vi "CustomPID_v2.1.vi"(0 "Kp":dbl, 1 "Process Variable":dbl, 2 "Goal":dbl, 5 "Ki":dbl, 7 "Kd":dbl, 9 "N-Diff":i32=3, 11 "N-Int":i32=12, 12 "Reinit":bool, 13 "Max Ouput":dbl=1.0, 14 "Min Output":dbl=-1.0) -> (4 "Current Error":dbl, 8 "Command":dbl, 15 "PID Tracking":T1(graph))   [LabVIEW 2016]
uses:
  <vilib>/Analysis/NI_AALPro.lvlib
panel:
  out "x-y":u32
  out "Absolute Iterations":i32
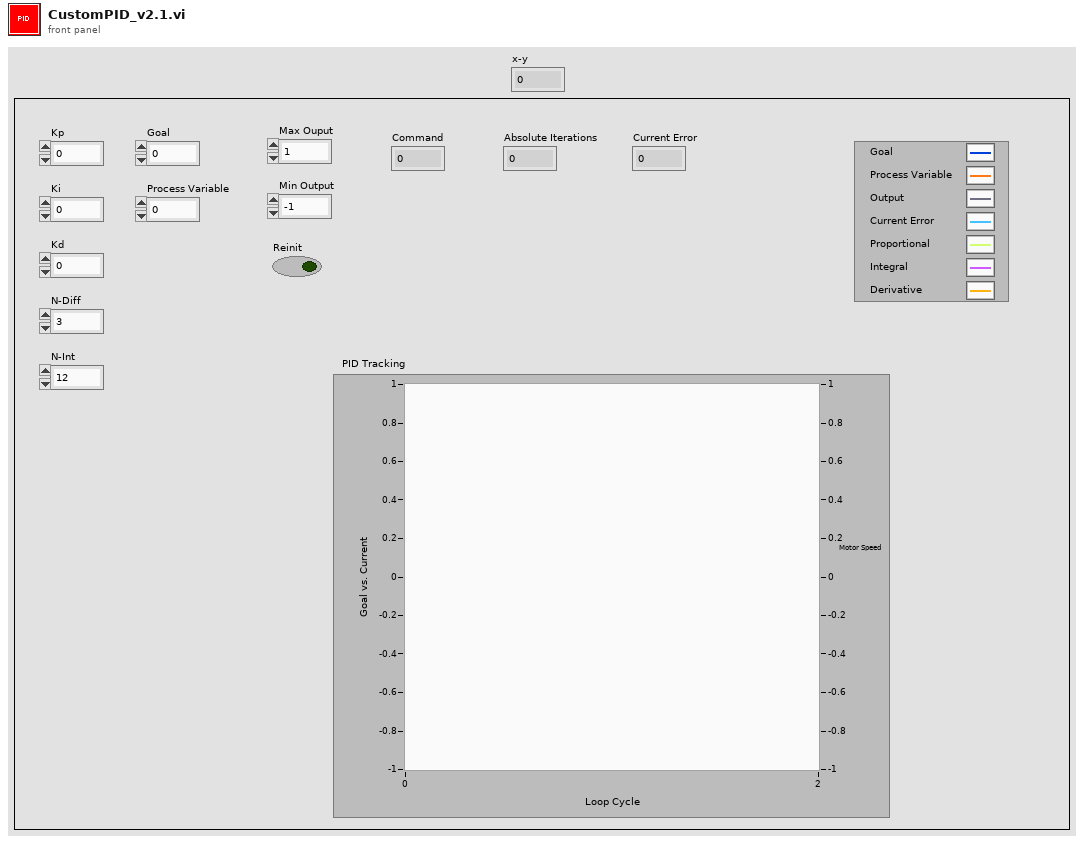
[diagram p1: front panel]
types:
  T1 = cluster{"Goal":dbl, "Process Variable":dbl, "Max Ouput":dbl, dbl, dbl, dbl, dbl}
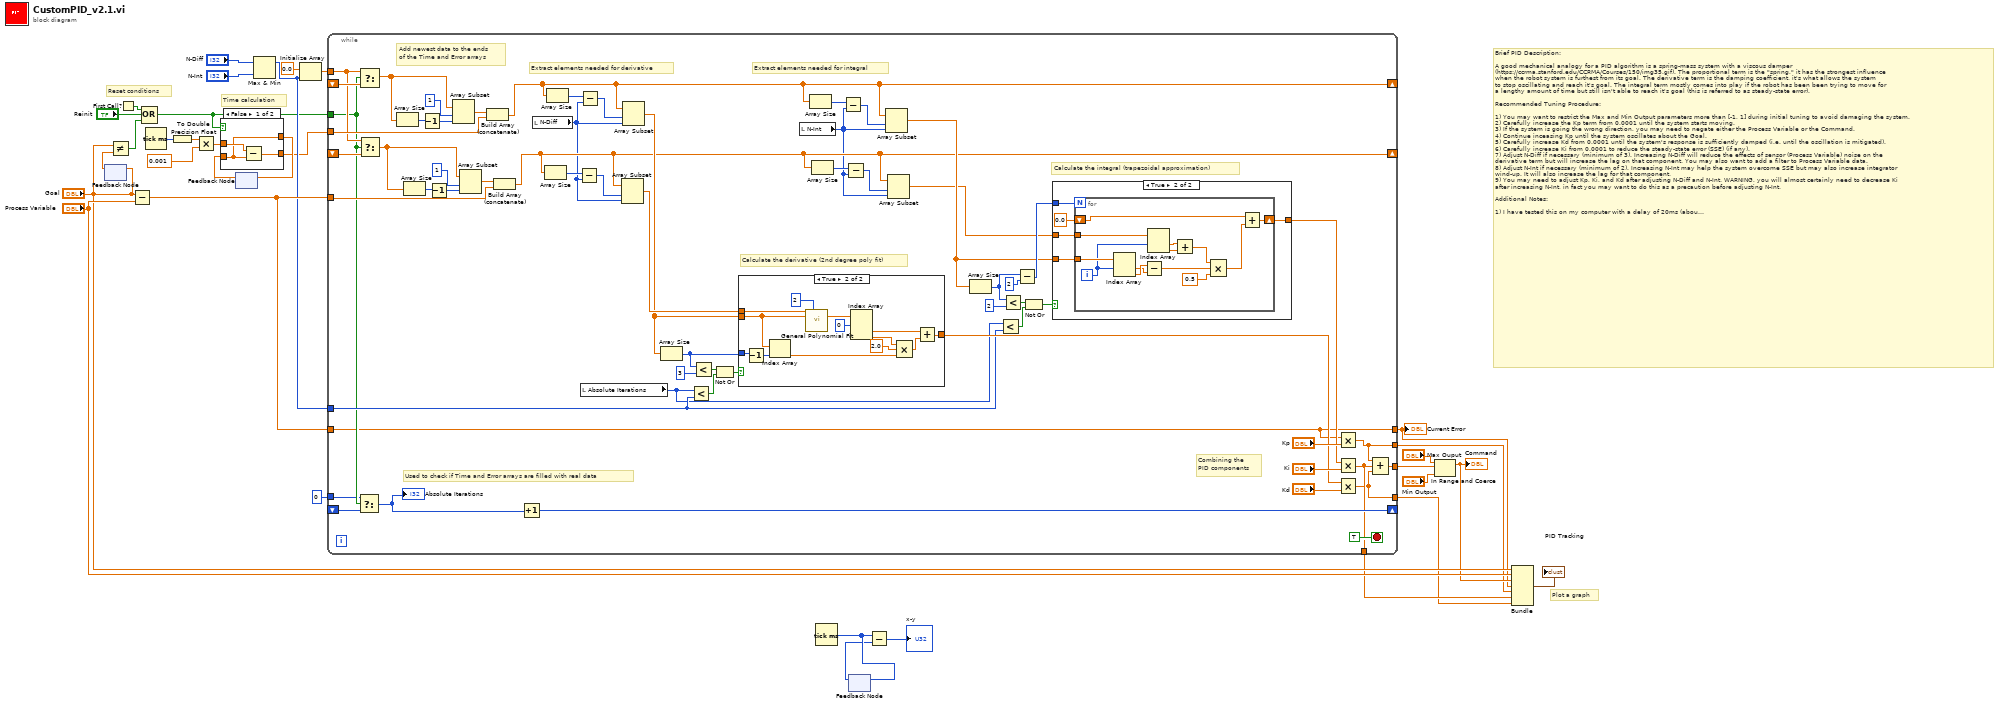
[diagram p0: block diagram]
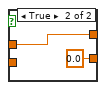
[diagram p2: hidden frame]
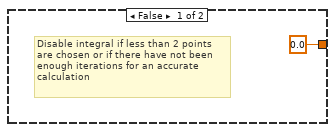
[diagram p3: hidden frame]
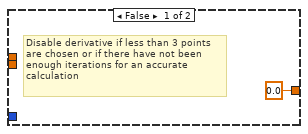
[diagram p4: hidden frame]
diagram:
  # "Time calculation"
  # "Brief PID Description:\n\nA good mechanical analogy for a PID algorithm is a spring-mass system with a viscous damper \n(https://ccrma.stanford.edu/CCRMA/Courses/150/img35.gif). The proportional term is the \"spring,\" it has the strongest influence\nwhen the robot system is furthest from its goal. The derivative term is the damping coefficient, it's what allows the system\nto stop oscillating and reach it's goal. The integral term mostly comes into play if the robot has been been trying to move for \na lengthy amount of time but still isn't able to reach it's goal (this is referred to as steady-state error).\n\nRecommended Tuning Procedure:\n\n1) You may want to restrict the Max and Min Output parameters more than [-1, 1] during initial tuning to avoid damaging the system.\n2) Carefully increase the Kp term from 0.0001 until the system starts moving.\n3) If the system is going the wrong direction, you may need to negate either the Process Variable or the Command.\n4) Continue inceasing Kp until the system oscillates about the Goal.\n5) Carefully increase Kd from 0.0001 until the system's response is sufficiently damped (i.e. until the oscillation is mitigated).\n6) Carefully increase Ki from 0.0001 to reduce the steady-state error (SSE) (if any).\n7) Adjust N-Diff if necessary (minimum of 3). Increasing N-Diff will reduce the effects of sensor (Process Variable) noise on the \nderivative term but will increase the lag on that component. You may also want to add a filter to Process Variable data.\n8) Adjust N-Int if necessary (minimum of 2). Increasing N-Int may help the system overcome SSE but may also increase integrator\nwind-up. It will also increase the lag for that component.\n9) You may need to adjust Kp, Ki, and Kd after adjusting N-Diff and N-Int. WARNING, you will almost certainly need to decrease Ki\nafter increasing N-Int, in fact you may want to do this as a precaution before adjusting N-Int. \n\nAdditional Notes:\n\n1) I have tested this on my computer with a delay of 20ms (about what I expect for the robot) and it appears to function correctly.\nThat being said I have NOT tested this on an actual, physical system. So exercise caution when testing it for the first time.\n2) Make sure that execution type for all instances of this VI are set to \"preallocated clone reentrant execution.\"\n3) Several parts of this VI were inspired by a PID algorithm written by Dr. Ira Hill at the University of Florida.\n4) If you have any questions, feel free to contact me at lrscime@ufl.edu."
  # "Plot a graph"
  # "Reset conditions"
  n1 = feedback-in #1("Goal") -> ()
  n2 = feedback #1() -> (w20:dbl)  [unwired: 1 in]
  n3 = Not Equal?(x="Goal", y=w20) -> (x != y?=w19:bool)
  n4 = First Call?() -> (First Call?: T/F=w28:bool)
  n5 = Subtract(x="Goal", y="Process Variable") -> (x-y=w33:dbl)
  n6 = Compound Arithmetic op=OR(w28, "Reinit", w19) -> (w10:bool)
  n7 = Tick Count (ms)() -> (millisecond timer value=w17:u32)
  n8 = To Double Precision Float(number=w17) -> (double precision float=w16:dbl)
  n9 = Multiply(x=w16, y=0.001) -> (x*y=w14:dbl)
  n10 = feedback #2() -> (w12:dbl)  [unwired: 1 in]
  n11 = case shown="False" w10 {
    tunnel: w14 -> [w36 w38]
    tunnel: [w34 w38] -> w13
    tunnel: [w35 0.0] -> w11
    tunnel: w12 -> [w34 _]
    frame False {
      n12 = Subtract(x=w36, y=w34) -> (x-y=w35:dbl)
    }
    frame True {
    }
  }
  n13 = feedback-in #2(w13) -> ()
  n14 = Max & Min(x="N-Diff", y="N-Int") -> (max(x,y)=w22:i32)  [unwired: 1 out]
  n15 = Initialize Array(0.0 ("element"), w22) -> (w24:dbl[])
  n16 = while {
    tunnel: [w95] -> w31
    tunnel: w33 -> [w86]
    shift-right: [w70] -> _
    shift-left: _ -> [w55]
    tunnel: w11 -> [w90]
    shift-right: [w56] -> _
    shift-left: _ -> [w52]
    tunnel: w22 -> [w62]
    tunnel: w33 -> [w42]
    shift-right: [w63] -> _
    shift-left: _ -> [w49]
    tunnel: w10 -> [w48]
    tunnel: w24 -> [w53]
    tunnel: 0 -> [w44]
    tunnel: [w42] -> w7
    tunnel: [w41] -> w6
    tunnel: [w40] -> w5
    tunnel: [w39] -> w4
    stop <- TRUE stop-if-true
    # "Combining the\nPID components"
    # "Add newest data to the ends\nof the Time and Error arrays"
    # "Used to check if Time and Error arrays are filled with real data"
    # "Extract elements needed for integral"
    # "Extract elements needed for derivative"
    # "Calculate the integral (trapezoidal approximation)"
    # "Calculate the derivative (2nd degree poly fit)"
    n17 = Select(t=w44, s=w48, f=w49) -> (s? t:f=w50:i32)
    "Absolute Iterations" <- w50
    n18 = Select(t=w53, s=w48, f=w55) -> (s? t:f=w54:dbl[])
    n19 = Select(t=w53, s=w48, f=w52) -> (s? t:f=w51:dbl[])
    n20 = Array Size(array=w54) -> (size(s)=w93:i32)
    n21 = Array Size(array=w51) -> (size(s)=w88:i32)
    n22 = Decrement(x=w93) -> (x-1=w92:i32)
    n23 = Decrement(x=w88) -> (x-1=w87:i32)
    n24 = Array Subset(array=w54, index=1, length=w92) -> (w91:dbl[])
    n25 = Array Subset(array=w51, index=1, length=w87) -> (w85:dbl[])
    n26 = Build Array (concatenate)(w91, w90) -> (w70:dbl[])
    n27 = Build Array (concatenate)(w85, w86) -> (w56:dbl[])
    n28 = Increment(x=w50) -> (x+1=w63:i32)
    n29 = local read "N-Diff"() -> (w46:i32)
    n30 = Array Size(array=w56) -> (size(s)=w81:i32)
    n31 = Array Size(array=w70) -> (size(s)=w84:i32)
    n32 = Subtract(x=w81, y=w46) -> (x-y=w82:i32)
    n33 = Subtract(x=w84, y=w46) -> (x-y=w83:i32)
    n34 = local read "Absolute Iterations"() -> (w43:i32)
    n35 = Array Subset(array=w56, index=w82, length=w46) -> (w80:dbl[])
    n36 = Array Subset(array=w70, index=w83, length=w46) -> (w79:dbl[])
    n37 = Array Size(array=w79) -> (size(s)=w77:i32)
    n38 = Less?(x=w43, y=w62) -> (x < y?=w75:bool)
    n39 = Less?(x=w77, y=3) -> (x < y?=w78:bool)
    n40 = Not Or(1:w75, 2:w78) -> (0:w74:bool)
    n41 = case shown="True" w74 {
      tunnel: w80 -> [_ w125]
      tunnel: w77 -> [_ w124]
      tunnel: w79 -> [_ w122]
      tunnel: [0.0 w120] -> w73
      frame False {
        # "Disable derivative if less than 3 points \nare chosen or if there have not been \nenough iterations for an accurate \ncalculation"
      }
      frame True {
        n42 = Decrement(x=w124) -> (x-1=w123:i32)
        n43 = Index Array(array=w122, index=w123) -> (element=w121:dbl)
        n44 = call <vilib>:"General Polynomial Fit.vi"("Y"=w125, "polynomial order"=2, "X"=w122) -> ("Polynomial Coefficients"=w131:dbl[])  [unwired: 9 in, 3 out]
        n45 = Index Array(array=w131, index #1=0 ("index")) -> (element #2=w127:dbl, element #3=w129:dbl)  [unwired: 2 in, 1 out]
        n46 = Compound Arithmetic op=MULTIPLY(w129, 2.0 ("y"), w121) -> (w126:dbl)
        n47 = Add(x=w127, y=w126) -> (x+y=w120:dbl)
      }
    }
    n48 = local read "N-Int"() -> (w45:i32)
    n49 = Array Size(array=w70) -> (size(s)=w72:i32)
    n50 = Array Size(array=w56) -> (size(s)=w69:i32)
    n51 = Subtract(x=w72, y=w45) -> (x-y=w71:i32)
    n52 = Subtract(x=w69, y=w45) -> (x-y=w68:i32)
    n53 = Array Subset(array=w70, index=w71, length=w45) -> (w57:dbl[])
    n54 = Array Subset(array=w56, index=w68, length=w45) -> (w47:dbl[])
    n55 = Array Size(array=w57) -> (size(s)=w60:i32)
    n56 = Less?(x=w43, y=w62) -> (x < y?=w65:bool)
    n57 = Less?(x=w60, y=2) -> (x < y?=w67:bool)
    n58 = Subtract(x=w60, y=2) -> (x-y=w59:i32)
    n59 = Not Or(1:w65, 2:w67) -> (0:w64:bool)
    n60 = case shown="True" w64 {
      tunnel: [0.0 w103] -> w61
      tunnel: w59 -> [_ w105]
      tunnel: w57 -> [_ w102]
      tunnel: w47 -> [_ w101]
      frame False {
        # "Disable integral if less than 2 points \nare chosen or if there have not been \nenough iterations for an accurate \ncalculation"
      }
      frame True {
        n61 = for {
          N: w105 -> [_]
          shift-right: [w117] -> w103
          shift-left: 0.0 -> [w118]
          tunnel: w102 -> [w116]
          tunnel: w101 -> [w109]
          i -> [w110]
          n62 = Index Array(array=w116, index #1=w110) -> (element #1=w114:dbl, element #2=w115:dbl)  [unwired: 1 in]
          n63 = Subtract(x=w115, y=w114) -> (x-y=w113:dbl)
          n64 = Index Array(array=w109, index #1=w110) -> (element #1=w107:dbl, element #2=w108:dbl)  [unwired: 1 in]
          n65 = Add(x=w107, y=w108) -> (x+y=w106:dbl)
          n66 = Compound Arithmetic op=MULTIPLY(w106, w113, 0.5 ("value")) -> (w111:dbl)
          n67 = Add(x=w118, y=w111) -> (x+y=w117:dbl)
        }
      }
    }
    n68 = Multiply(x=w42, y="Kp") -> (x*y=w41:dbl)
    n69 = Multiply(x=w61, y="Ki") -> (x*y=w40:dbl)
    n70 = Multiply(x=w73, y="Kd") -> (x*y=w39:dbl)
    n71 = Compound Arithmetic op=ADD(w41, w40, w39) -> (w95:dbl)
  }
  "Current Error" <- w7
  n72 = Tick Count (ms)() -> (millisecond timer value=w3:u32)
  n73 = feedback-in #3(w3) -> ()
  n74 = feedback #3() -> (w2:u32)  [unwired: 1 in]
  n75 = Subtract(x=w3, y=w2) -> (x-y=→"x-y":u32)
  n76 = In Range and Coerce(upper limit="Max Ouput", x=w31, lower limit="Min Output") -> (coerced(x)=w9:dbl)  [unwired: 1 out]
  "Command" <- w9
  n77 = Bundle("Goal"="Goal", "Process Variable"="Process Variable", "Max Ouput"=w9, w7, w6, w5, w4) -> (→"PID Tracking":T1)  [unwired: 1 in]
